vi "Error Control.vi"(4 "Command":T1, 5 "error in (no error)":errorcluster, 8 "Source":string) -> (0 "error out":errorcluster)   [LabVIEW 2018]
doc: "[Ver 1.00]\nREUSEABLE COMPONENT\nDESCRIPTION\nReuseable Component\nDisplays or logs errors. \n\nCOMMANDS\nNo Command - Error :Throw the error dialog.\nSet to Dev Mode : This should be set first, when Set Error is called the dialog will be displayed. \nSet to Released Mode : This should be set first, when Set Error is called the error will be quietly filed away.\nSet Error : Throw or Log an error.\nLog Error : Log an error regardless of Mode.\nThrow Error : Throw dialog regardless of Mode.\nLog & Throw Error : Do both regardless of Mode.\n\nERROR HANDLING\nWill throw an error if No Command is set\n\n---------------------------------------------------------\nVERSION CONTROL\n1.00 New version SSDC 14/3/2000"
uses:
  ErrorCommand.ctl
  Controls/DisplayQCommand.ctl
  Error/ErrorMessage.ctl
panel:
  # "Input"
  # "Output"
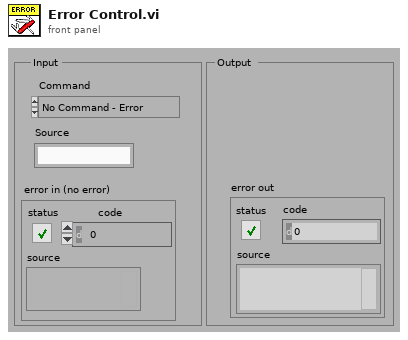
[diagram p1: front panel]
types:
  T1 = typedef "ErrorCommand.ctl" = enum16{"No Command - Error", "Set to Dev Mode", "Set To Released Mode", "Set Error", "Log Error", "Throw Error", "Log & Throw Error", "Set Error Timed"}
  T2 = typedef "ErrorMessage.ctl" = enum16{"No Message - Ignore", "Display Message", "Stop"}
  T3 = typedef "DisplayQCommand.ctl" = enum16{"No Command - Error", "Initialise", "Get Q Reference", "Add Item to Bottom", "Add Item to Top", "Flush Q", "Dequeue", "Peek Next Element", "Close"}
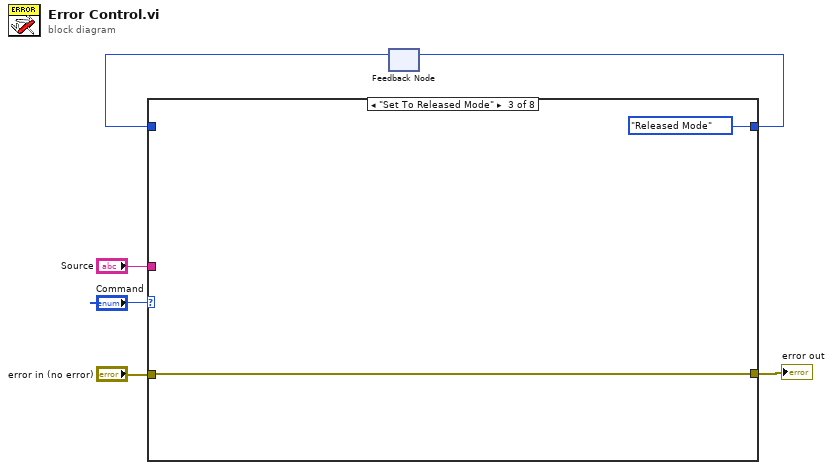
[diagram p0: block diagram]
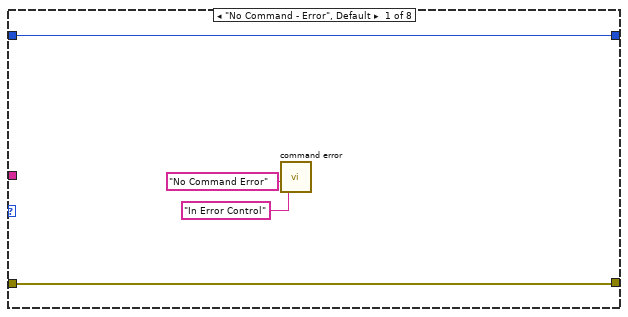
[diagram p2: hidden frame]
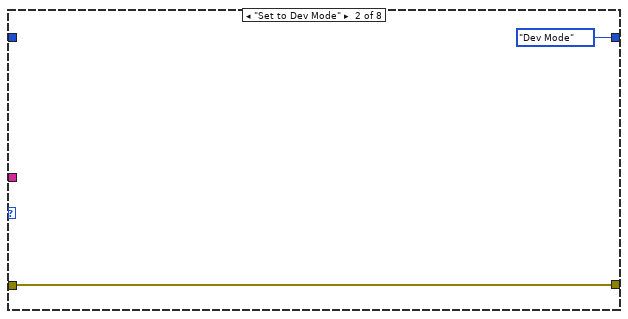
[diagram p3: hidden frame]
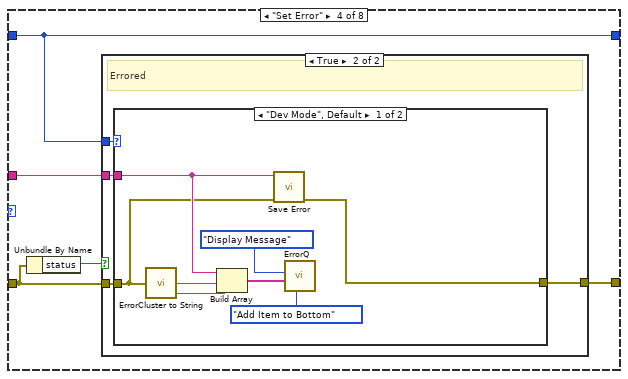
[diagram p4: hidden frame]
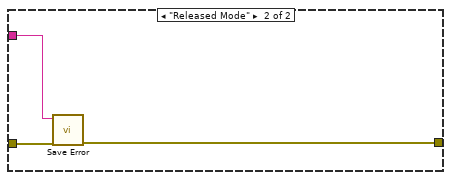
[diagram p6: hidden frame]
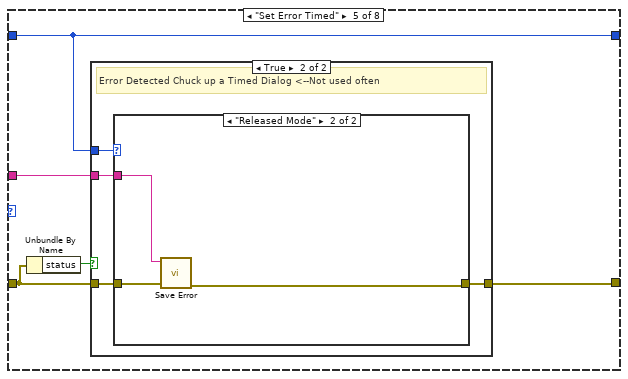
[diagram p7: hidden frame]
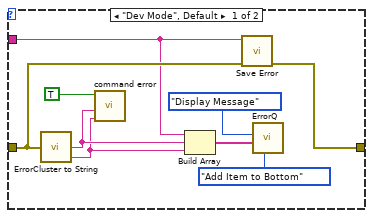
[diagram p9: hidden frame]
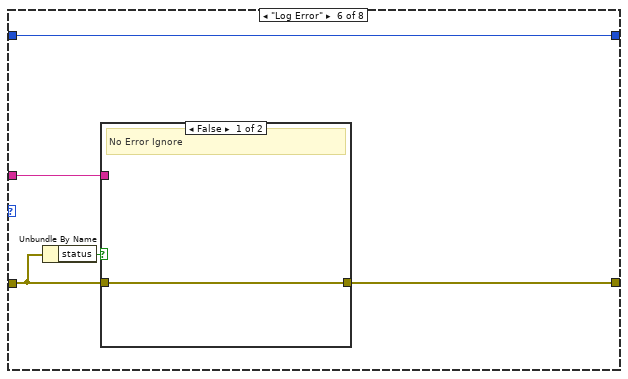
[diagram p10: hidden frame]
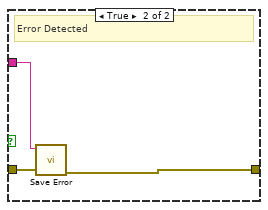
[diagram p11: hidden frame]
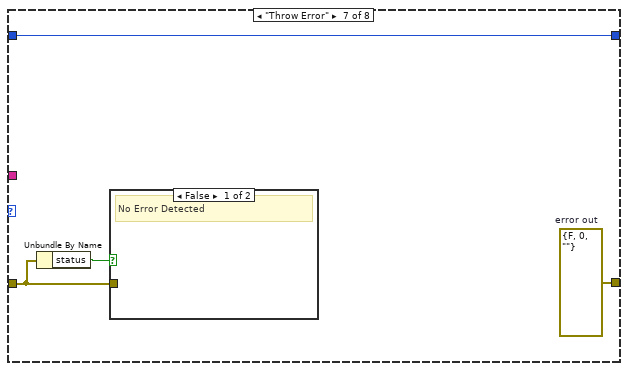
[diagram p12: hidden frame]
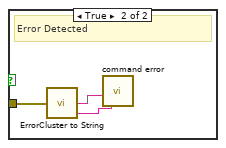
[diagram p13: hidden frame]
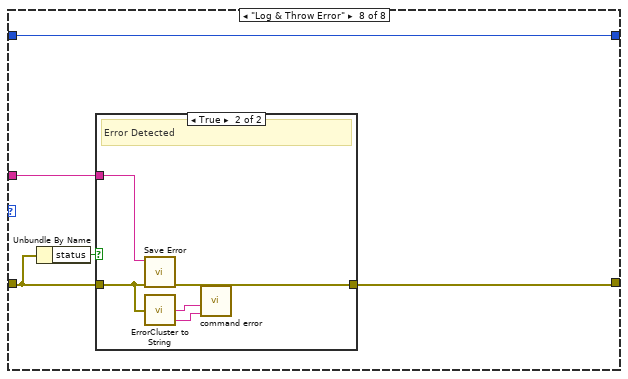
[diagram p14: hidden frame]
diagram:
  n1 = feedback #1() -> (w2:enum16{"Dev Mode", "Released Mode"})  [unwired: 1 in]
  n2 = case shown="\"Set To Released Mode\"" "Command" {
    tunnel: [w10 enum16{"Dev Mode", "Released Mode"}."Dev Mode" enum16{"Dev Mode", "Released Mode"}."Released Mode" w19 w40 w62 w70 w78] -> w3
    tunnel: w2 -> [w10 _ _ w19 w40 w62 w70 w78]
    tunnel: "error in (no error)" -> [w7 w11 w13 w18 w39 w60 w68 w76]
    tunnel: "Source" -> [_ _ _ w16 w36 w58 _ w75]
    tunnel: [w7 w11 w13 w15 w37 w59 w67 w74] -> w1
    frame "No Command - Error", Default {
      n3 = call "command error.vi"("Error Details"="In Error Control", "Comment"="No Command Error") -> ()  [unwired: 6 in]
    }
    frame "Set to Dev Mode" {
    }
    frame "Set To Released Mode" {
    }
    frame "Set Error" {
      n4 = Unbundle By Name(w18) -> ("status"=w17:bool)
      n5 = case shown="True" w17 {
        tunnel: w19 -> [_ w24]
        tunnel: w18 -> [w20 w23]
        tunnel: w16 -> [_ w22]
        tunnel: [w20 w21] -> w15
        frame False {
          # "No Error Ignore"
        }
        frame True {
          # "Errored"
          n6 = case shown="\"Dev Mode\", Default" w24 {
            tunnel: w23 -> [w26 w35]
            tunnel: w22 -> [w27 w33]
            tunnel: [w25 w34] -> w21
            frame "Dev Mode", Default {
              n7 = call "ErrorCluster to String.vi"("error in (no error)"=w26) -> ("ErrorMSG"=w30:string, "String"=w29:string)  [unwired: 3 in]
              n8 = Build Array(w27, w29, w30) -> (w28:string[])
              n9 = call "Save Error.vi"("Error In (no error)"=w26, "Source"=w27) -> ("error out"=w25:errorcluster)  [unwired: 5 in]
              n10 = call "ErrorQ.vi"("command"=DisplayQCommand."Add Item to Bottom", "DataIn"=w28, "ErrorMessage"=ErrorMessage."Display Message") -> ()  [unwired: 2 in, 4 out]
            }
            frame "Released Mode" {
              n11 = call "Save Error.vi"("Error In (no error)"=w35, "Source"=w33) -> ("error out"=w34:errorcluster)  [unwired: 5 in]
            }
          }
        }
      }
    }
    frame "Set Error Timed" {
      n12 = Unbundle By Name(w39) -> ("status"=w38:bool)
      n13 = case shown="True" w38 {
        tunnel: w40 -> [_ w45]
        tunnel: w39 -> [w41 w44]
        tunnel: [w41 w43] -> w37
        tunnel: w36 -> [_ w42]
        frame False {
          # "No Error"
        }
        frame True {
          # "Error Detected Chuck up a Timed Dialog <--Not used often"
          n14 = case shown="\"Released Mode\"" w45 {
            tunnel: w44 -> [w49 w57]
            tunnel: [w50 w55] -> w43
            tunnel: w42 -> [w48 w56]
            frame "Dev Mode", Default {
              n15 = call "ErrorCluster to String.vi"("error in (no error)"=w49) -> ("ErrorMSG"=w46:string, "String"=w47:string)  [unwired: 3 in]
              n16 = call "command error.vi"("Error Details"=w46, "Comment"=w47, "5 Sec Countdown"=TRUE) -> ()  [unwired: 5 in]
              n17 = Build Array(w48, w47, w46) -> (w51:string[])
              n18 = call "Save Error.vi"("Error In (no error)"=w49, "Source"=w48) -> ("error out"=w50:errorcluster)  [unwired: 5 in]
              n19 = call "ErrorQ.vi"("command"=DisplayQCommand."Add Item to Bottom", "DataIn"=w51, "ErrorMessage"=ErrorMessage."Display Message") -> ()  [unwired: 2 in, 4 out]
            }
            frame "Released Mode" {
              n20 = call "Save Error.vi"("Error In (no error)"=w57, "Source"=w56) -> ("error out"=w55:errorcluster)  [unwired: 5 in]
            }
          }
        }
      }
    }
    frame "Log Error" {
      n21 = Unbundle By Name(w60) -> ("status"=w61:bool)
      n22 = case shown="False" w61 {
        tunnel: w60 -> [w63 w66]
        tunnel: [w63 w65] -> w59
        tunnel: w58 -> [_ w64]
        frame False {
          # "No Error Ignore"
        }
        frame True {
          # "Error Detected"
          n23 = call "Save Error.vi"("Error In (no error)"=w66, "Source"=w64) -> ("error out"=w65:errorcluster)  [unwired: 5 in]
        }
      }
    }
    frame "Throw Error" {
      w67 = errorcluster {"status"=FALSE, "code"=0, "source"=""}  # error out
      n24 = Unbundle By Name(w68) -> ("status"=w69:bool)
      n25 = case shown="False" w69 {
        tunnel: w68 -> [_ w73]
        frame False {
          # "No Error Detected"
        }
        frame True {
          # "Error Detected"
          n26 = call "ErrorCluster to String.vi"("error in (no error)"=w73) -> ("ErrorMSG"=w71:string, "String"=w72:string)  [unwired: 3 in]
          n27 = call "command error.vi"("Error Details"=w71, "Comment"=w72) -> ()  [unwired: 6 in]
        }
      }
    }
    frame "Log & Throw Error" {
      n28 = Unbundle By Name(w76) -> ("status"=w77:bool)
      n29 = case shown="True" w77 {
        tunnel: w76 -> [w79 w82]
        tunnel: w75 -> [_ w81]
        tunnel: [w79 w80] -> w74
        frame False {
          # "No Error Detected"
        }
        frame True {
          # "Error Detected"
          n30 = call "Save Error.vi"("Error In (no error)"=w82, "Source"=w81) -> ("error out"=w80:errorcluster)  [unwired: 5 in]
          n31 = call "ErrorCluster to String.vi"("error in (no error)"=w82) -> ("ErrorMSG"=w83:string, "String"=w84:string)  [unwired: 3 in]
          n32 = call "command error.vi"("Error Details"=w83, "Comment"=w84) -> ()  [unwired: 6 in]
        }
      }
    }
  }
  "error out" <- w1
  n33 = feedback-in #1(w3) -> ()
